vi "rsidr_core_global.vi"() -> ()   [LabVIEW 2015, in "Rohde&Schwarz CMXP GPRF.lvlib"] (continued)
ARB File All Names", "Data Type"=6, "Command"="SOUR:GPRF:GEN{instance}:SEQ:APO:WAV:ALL?", "Access"=0, "Range Table"="", "Read Callback"="", "Write Callback"="", "Supported Models"="", "Instrument Options"="", "Flags"=0, "Help"="Queries the names of the ARB files in the file pool.\n\nAvailable Repeated Capabilities:\ninstance: i0, i1, i2, i3, i4, i5, i6, i7, i8, i9, i10, i11, i12, i13, i14, i15, i16, i17, i18, i19, i20, i21, i22, i23, i24, i25, i26, i27, i28, i29, i30, i31, i32\r\n\nRemote-control command(s):\nSOURce:GPRF:GEN<i>:SEQuencer:APOol:WAVeform:ALL?"}, {"Level"=4, "Class Only"=FALSE, "Identifier"="RSCMXPGPRF_ATTR_HIDDEN_SEQUENCER_ARB_FILE_SAMPLE_RATE", "Descriptive Name"="Sequencer ARB File Sample Rate", "Data Type"=1, "Command"="SOUR:GPRF:GEN{instance}:SEQ:APO:SRAT?", "Access"=0, "Range Table"="", "Read Callback"="", "Write Callback"="", "Supported Models"="", "Instrument Options"="", "Flags"=8, "Help"="Queries the sample rate of the ARB file with the specified <Index>.\n\nAvailable Repeated Capabilities:\ninstance: i0, i1, i2, i3, i4, i5, i6, i7, i8, i9, i10, i11, i12, i13, i14, i15, i16, i17, i18, i19, i20, i21, i22, i23, i24, i25, i26, i27, i28, i29, i30, i31, i32\r\n\nRemote-control command(s):\nSOURce:GPRF:GEN<i>:SEQuencer:APOol:SRATe?"}, {"Level"=4, "Class Only"=FALSE, "Identifier"="RSCMXPGPRF_ATTR_SEQUENCER_ARB_FILE_ALL_SAMPLE_RATES", "Descriptive Name"="Sequencer ARB File All Sample Rates", "Data Type"=6, "Command"="SOUR:GPRF:GEN{instance}:SEQ:APO:SRAT:ALL?", "Access"=0, "Range Table"="", "Read Callback"="", "Write Callback"="", "Supported Models"="", "Instrument Options"="", "Flags"=0, "Help"="Queries the sample rates of the ARB files in the file pool.\n\nAvailable Repeated Capabilities:\ninstance: i0, i1, i2, i3, i4, i5, i6, i7, i8, i9, i10, i11, i12, i13, i14, i15, i16, i17, i18, i19, i20, i21, i22, i23, i24, i25, i26, i27, i28, i29, i30, i31, i32\r\n\nRemote-control command(s):\nSOURce:GPRF:GEN<i>:SEQuencer:APOol:SRATe:ALL?"}, {"Level"=4, "Class Only"=FALSE, "Identifier"="RSCMXPGPRF_ATTR_HIDDEN_SEQUENCER_ARB_FILE_NUMBER_OF_SAMPLES", "Descriptive Name"="Sequencer ARB File Number Of Samples", "Data Type"=0, "Command"="SOUR:GPRF:GEN{instance}:SEQ:APO:SAMP?", "Access"=0, "Range Table"="", "Read Callback"="", "Write Callback"="", "Supported Models"="", "Instrument Options"="", "Flags"=8, "Help"="Queries the number of samples in the ARB file with the specified <Index>.\n\nAvailable Repeated Capabilities:\ninstance: i0, i1, i2, i3, i4, i5, i6, i7, i8, i9, i10, i11, i12, i13, i14, i15, i16, i17, i18, i19, i20, i21, i22, i23, i24, i25, i26, i27, i28, i29, i30, i31, i32\r\n\nRemote-control command(s):\nSOURce:GPRF:GEN<i>:SEQuencer:APOol:SAMPles?"}, {"Level"=4, "Class Only"=FALSE, "Identifier"="RSCMXPGPRF_ATTR_SEQUENCER_ARB_FILE_ALL_NUMBERS_OF_SAMPLES", "Descriptive Name"="Sequencer ARB File All Numbers Of Samples", "Data Type"=6, "Command"="SOUR:GPRF:GEN{instance}:SEQ:APO:SAMP:ALL?", "Access"=0, "Range Table"="", "Read Callback"="", "Write Callback"="", "Supported Models"="", "Instrument Options"="", "Flags"=0, "Help"="Queries the numbers of samples in the ARB files of the file pool.\n\nAvailable Repeated Capabilities:\ninstance: i0, i1, i2, i3, i4, i5, i6, i7, i8, i9, i10, i11, i12, i13, i14, i15, i16, i17, i18, i19, i20, i21, i22, i23, i24, i25, i26, i27, i28, i29, i30, i31, i32\r\n\nRemote-control command(s):\nSOURce:GPRF:GEN<i>:SEQuencer:APOol:SAMPles:ALL?"}, {"Level"=4, "Class Only"=FALSE, "Identifier"="RSCMXPGPRF_ATTR_HIDDEN_SEQUENCER_ARB_FILE_DURATION", "Descriptive Name"="Sequencer ARB File Duration", "Data Type"=1, "Command"="SOUR:GPRF:GEN{instance}:SEQ:APO:DUR?", "Access"=0, "Range Table"="", "Read Callback"="", "Write Callback"="", "Supported Models"="", "Instrument Options"="", "Flags"=8, "Help"="Queries the duration of the ARB file with the specified <Index>.\n\nAvailable Repeated Capabilities:\ninstance: i0, i1, i2, i3, i4, i5, i6, i7, i8, i9, i10, i11, i12, i13, i14, i15, i16, i17, i18, i19, i20, i21, i22, i23, i24, i25, i26, i27, i28, i29, i30, i31, i32\r\n\nRemote-control command(s):\nSOURce:GPRF:GEN<i>:SEQuencer:APOol:DURation?"}, {"Level"=4, "Class Only"=FALSE, "Identifier"="RSCMXPGPRF_ATTR_SEQUENCER_ARB_FILE_ALL_DURATIONS", "Descriptive Name"="Sequencer ARB File All Durations", "Data Type"=6, "Command"="SOUR:GPRF:GEN{instance}:SEQ:APO:DUR:ALL?", "Access"=0, "Range Table"="", "Read Callback"="", "Write Callback"="", "Supported Models"="", "Instrument Options"="", "Flags"=0, "Help"="Queries the durations of the ARB files in the file pool.\n\nAvailable Repeated Capabilities:\ninstance: i0, i1, i2, i3, i4, i5, i6, i7, i8, i9, i10, i11, i12, i13, i14, i15, i16, i17, i18, i19, i20, i21, i22, i23, i24, i25, i26, i27, i28, i29, i30, i31, i32\r\n\nRemote-control command(s):\nSOURce:GPRF:GEN<i>:SEQuencer:APOol:DURation:ALL?"}, {"Level"=4, "Class Only"=FALSE, "Identifier"="RSCMXPGPRF_ATTR_HIDDEN_SEQUENCER_ARB_FILE_REQ_OPTIONS", "Descriptive Name"="Sequencer ARB File Req Options", "Data Type"=2, "Command"="SOUR:GPRF:GEN{instance}:SEQ:APO:ROPT?", "Access"=0, "Range Table"="", "Read Callback"="", "Write Callback"="", "Supported Models"="", "Instrument Options"="", "Flags"=8, "Help"="Queries the options required by the ARB file with the specified <Index>.\n\nAvailable Repeated Capabilities:\ninstance: i0, i1, i2, i3, i4, i5, i6, i7, i8, i9, i10, i11, i12, i13, i14, i15, i16, i17, i18, i19, i20, i21, i22, i23, i24, i25, i26, i27, i28, i29, i30, i31, i32\r\n\nRemote-control command(s):\nSOURce:GPRF:GEN<i>:SEQuencer:APOol:ROPTion?"}, {"Level"=4, "Class Only"=FALSE, "Identifier"="RSCMXPGPRF_ATTR_SEQUENCER_ARB_FILE_ALL_REQ_OPTIONS", "Descriptive Name"="Sequencer ARB File All Req Options", "Data Type"=6, "Command"="SOUR:GPRF:GEN{instance}:SEQ:APO:ROPT:ALL?", "Access"=0, "Range Table"="", "Read Callback"="", "Write Callback"="", "Supported Models"="", "Instrument Options"="", "Flags"=0, "Help"="Queries the options required by the ARB files in the file pool.\n\nAvailable Repeated Capabilities:\ninstance: i0, i1, i2, i3, i4, i5, i6, i7, i8, i9, i10, i11, i12, i13, i14, i15, i16, i17, i18, i19, i20, i21, i22, i23, i24, i25, i26, i27, i28, i29, i30, i31, i32\r\n\nRemote-control command(s):\nSOURce:GPRF:GEN<i>:SEQuencer:APOol:ROPTion:ALL?"}, {"Level"=4, "Class Only"=FALSE, "Identifier"="RSCMXPGPRF_ATTR_HIDDEN_SEQUENCER_ARB_FILE_PEAK_OFFSETS", "Descriptive Name"="Sequencer ARB File Peak Offsets", "Data Type"=1, "Command"="SOUR:GPRF:GEN{instance}:SEQ:APO:POFF?", "Access"=0, "Range Table"="", "Read Callback"="", "Write Callback"="", "Supported Models"="", "Instrument Options"="", "Flags"=8, "Help"="Queries the peak offset of the ARB file with the specified <Index>.\n\nAvailable Repeated Capabilities:\ninstance: i0, i1, i2, i3, i4, i5, i6, i7, i8, i9, i10, i11, i12, i13, i14, i15, i16, i17, i18, i19, i20, i21, i22, i23, i24, i25, i26, i27, i28, i29, i30, i31, i32\r\n\nRemote-control command(s):\nSOURce:GPRF:GEN<i>:SEQuencer:APOol:POFFset?"}, {"Level"=4, "Class Only"=FALSE, "Identifier"="RSCMXPGPRF_ATTR_SEQUENCER_ARB_FILE_ALL_PEAK_OFFSETS", "Descriptive Name"="Sequencer ARB File All Peak Offsets", "Data Type"=6, "Command"="SOUR:GPRF:GEN{instance}:SEQ:APO:POFF:ALL?", "Access"=0, "Range Table"="", "Read Callback"="", "Write Callback"="", "Supported Models"="", "Instrument Options"="", "Flags"=0, "Help"="Queries the peak offsets of the ARB files in the file pool.\n\nAvailable Repeated Capabilities:\ninstance: i0, i1, i2, i3, i4, i5, i6, i7, i8, i9, i10, i11, i12, i13, i14, i15, i16, i17, i18, i19, i20, i21, i22, i23, i24, i25, i26, i27, i28, i29, i30, i31, i32\r\n\nRemote-control command(s):\nSOURce:GPRF:GEN<i>:SEQuencer:APOol:POFFset:ALL?"}, {"Level"=4, "Class Only"=FALSE, "Identifier"="RSCMXPGPRF_ATTR_HIDDEN_SEQUENCER_ARB_FILE_PEAK_TO_AVG_RATIO", "Descriptive Name"="Sequencer ARB File Peak To Avg Ratio", "Data Type"=1, "Command"="SOUR:GPRF:GEN{instance}:SEQ:APO:PAR?", "Access"=0, "Range Table"="", "Read Callback"="", "Write Callback"="", "Supported Models"="", "Instrument Options"="", "Flags"=8, "Help"="Queries the peak to average ratio of the ARB file with the specified <Index>.\n\nAvailable Repeated Capabilities:\ninstance: i0, i1, i2, i3, i4, i5, i6, i7, i8, i9, i10, i11, i12, i13, i14, i15, i16, i17, i18, i19, i20, i21, i22, i23, i24, i25, i26, i27, i28, i29, i30, i31, i32\r\n\nRemote-control command(s):\nSOURce:GPRF:GEN<i>:SEQuencer:APOol:PARatio?"}, {"Level"=4, "Class Only"=FALSE, "Identifier"="RSCMXPGPRF_ATTR_SEQUENCER_ARB_FILE_ALL_PEAK_TO_AVG_RATIOS", "Descriptive Name"="Sequencer ARB File All Peak To Avg Ratios", "Data Type"=6, "Command"="SOUR:GPRF:GEN{instance}:SEQ:APO:PAR:ALL?", "Access"=0, "Range Table"="", "Read Callback"="", "Write Callback"="", "Supported Models"="", "Instrument Options"="", "Flags"=0, "Help"="Queries the peak to average ratios of the ARB files in the file pool.\n\nAvailable Repeated Capabilities:\ninstance: i0, i1, i2, i3, i4, i5, i6, i7, i8, i9, i10, i11, i12, i13, i14, i15, i16, i17, i18, i19, i20, i21, i22, i23, i24, i25, i26, i27, i28, i29, i30, i31, i32\r\n\nRemote-control command(s):\nSOURce:GPRF:GEN<i>:SEQuencer:APOol:PARatio:ALL?"}, {"Level"=4, "Class Only"=FALSE, "Identifier"="RSCMXPGPRF_ATTR_HIDDEN_SEQUENCER_ARB_FILE_CRC_PROTECTION", "Descriptive Name"="Sequencer ARB File CRC Protection", "Data Type"=0, "Command"="SOUR:GPRF:GEN{instance}:SEQ:APO:CRCP?", "Access"=0, "Range Table"="rsCmxpGprf_rngNoYesNav", "Read Callback"="", "Write Callback"="", "Supported Models"="", "Instrument Options"="", "Flags"=8, "Help"="Queries whether the ARB file with the specified <Index> contains a CRC checksum.\n\nAvailable Repeated Capabilities:\ninstance: i0, i1, i2, i3, i4, i5, i6, i7, i8, i9, i10, i11, i12, i13, i14, i15, i16, i17, i18, i19, i20, i21, i22, i23, i24, i25, i26, i27, i28, i29, i30, i31, i32\r\n\nRemote-control command(s):\nSOURce:GPRF:GEN<i>:SEQuencer:APOol:CRCProtect?"}, {"Level"=4, "Class Only"=FALSE, "Identifier"="RSCMXPGPRF_ATTR_SEQUENCER_ARB_FILE_ALL_CRC_PROTECTIONS", "Descriptive Name"="Sequencer ARB File All CRC Protections", "Data Type"=6, "Command"="SOUR:GPRF:GEN{instance}:SEQ:APO:CRCP:ALL?", "Access"=0, "Range Table"="", "Read Callback"="", "Write Callback"="", "Supported Models"="", "Instrument Options"="", "Flags"=0, "Help"="Queries whether the ARB files in the file pool contain CRC checksums.\n\nAvailable Repeated Capabilities:\ninstance: i0, i1, i2, i3, i4, i5, i6, i7, i8, i9, i10, i11, i12, i13, i14, i15, i16, i17, i18, i19, i20, i21, i22, i23, i24, i25, i26, i27, i28, i29, i30, i31, i32\r\n\nRemote-control command(s):\nSOURce:GPRF:GEN<i>:SEQuencer:APOol:CRCProtect:ALL?"}, {"Level"=4, "Class Only"=FALSE, "Identifier"="RSCMXPGPRF_ATTR_HIDDEN_SEQUENCER_ARB_FILE_RELIABILITY_INDICATOR", "Descriptive Name"="Sequencer ARB File Reliability Indicator", "Data Type"=0, "Command"="SOUR:GPRF:GEN{instance}:SEQ:APO:REL?", "Access"=0, "Range Table"="", "Read Callback"="", "Write Callback"="", "Supported Models"="", "Instrument Options"="", "Flags"=8, "Help"="Queries the reliability indicator for the ARB file with the specified <Index>.\n\nAvailable Repeated Capabilities:\ninstance: i0, i1, i2, i3, i4, i5, i6, i7, i8, i9, i10, i11, i12, i13, i14, i15, i16, i17, i18, i19, i20, i21, i22, i23, i24, i25, i26, i27, i28, i29, i30, i31, i32\r\n\nRemote-control command(s):\nSOURce:GPRF:GEN<i>:SEQuencer:APOol:RELiability?"}, {"Level"=4, "Class Only"=FALSE, "Identifier"="RSCMXPGPRF_ATTR_SEQUENCER_ARB_FILE_ALL_RELIABILITY_INDICATORS", "Descriptive Name"="Sequencer ARB File All Reliability Indicators", "Data Type"=6, "Command"="SOUR:GPRF:GEN{instance}:SEQ:APO:REL:ALL?", "Access"=0, "Range Table"="", "Read Callback"="", "Write Callback"="", "Supported Models"="", "Instrument Options"="", "Flags"=0, "Help"="Queries the reliability indicators for all ARB files in the file pool.\n\nAvailable Repeated Capabilities:\ninstance: i0, i1, i2, i3, i4, i5, i6, i7, i8, i9, i10, i11, i12, i13, i14, i15, i16, i17, i18, i19, i20, i21, i22, i23, i24, i25, i26, i27, i28, i29, i30, i31, i32\r\n\nRemote-control command(s):\nSOURce:GPRF:GEN<i>:SEQuencer:APOol:RELiability:ALL?"}, {"Level"=4, "Class Only"=FALSE, "Identifier"="RSCMXPGPRF_ATTR_HIDDEN_SEQUENCER_ARB_FILE_RELIABILITY_MESSAGE", "Descriptive Name"="Sequencer ARB File Reliability Message", "Data Type"=2, "Command"="SOUR:GPRF:GEN{instance}:SEQ:APO:RMES?", "Access"=0, "Range Table"="", "Read Callback"="", "Write Callback"="", "Supported Models"="", "Instrument Options"="", "Flags"=8, "Help"="Queries the reliability message for the ARB file with the specified <Index>.\n\nAvailable Repeated Capabilities:\ninstance: i0, i1, i2, i3, i4, i5, i6, i7, i8, i9, i10, i11, i12, i13, i14, i15, i16, i17, i18, i19, i20, i21, i22, i23, i24, i25, i26, i27, i28, i29, i30, i31, i32\r\n\nRemote-control command(s):\nSOURce:GPRF:GEN<i>:SEQuencer:APOol:RMESsage?"}, {"Level"=4, "Class Only"=FALSE, "Identifier"="RSCMXPGPRF_ATTR_SEQUENCER_ARB_FILE_ALL_RELIABILITY_MESSAGES", "Descriptive Name"="Sequencer ARB File All Reliability Messages", "Data Type"=6, "Command"="SOUR:GPRF:GEN{instance}:SEQ:APO:RMES:ALL?", "Access"=0, "Range Table"="", "Read Callback"="", "Write Callback"="", "Supported Models"="", "Instrument Options"="", "Flags"=0, "Help"="Queries the reliability messages for all ARB files in the file pool.\n\nAvailable Repeated Capabilities:\ninstance: i0, i1, i2, i3, i4, i5, i6, i7, i8, i9, i10, i11, i12, i13, i14, i15, i16, i17, i18, i19, i20, i21, i22, i23, i24, i25, i26, i27, i28, i29, i30, i31, i32\r\n\nRemote-control command(s):\nSOURce:GPRF:GEN<i>:SEQuencer:APOol:RMESsage:ALL?"}, {"Level"=4, "Class Only"=FALSE, "Identifier"="RSCMXPGPRF_ATTR_HIDDEN_SEQUENCER_ARB_FILE_PATH", "Descriptive Name"="Sequencer ARB File Path", "Data Type"=2, "Command"="SOUR:GPRF:GEN{instance}:SEQ:APO:PATH?", "Access"=0, "Range Table"="", "Read Callback"="", "Write Callback"="", "Supported Models"="", "Instrument Options"="", "Flags"=8, "Help"="Queries the path and file name of the ARB file with the specified <Index>.\n\nAvailable Repeated Capabilities:\ninstance: i0, i1, i2, i3, i4, i5, i6, i7, i8, i9, i10, i11, i12, i13, i14, i15, i16, i17, i18, i19, i20, i21, i22, i23, i24, i25, i26, i27, i28, i29, i30, i31, i32\r\n\nRemote-control command(s):\nSOURce:GPRF:GEN<i>:SEQuencer:APOol:PATH?"}, {"Level"=4, "Class Only"=FALSE, "Identifier"="RSCMXPGPRF_ATTR_SEQUENCER_ARB_FILE_ALL_PATHS", "Descriptive Name"="Sequencer ARB File All Paths", "Data Type"=6, "Command"="SOUR:GPRF:GEN{instance}:SEQ:APO:PATH:ALL?", "Access"=0, "Range Table"="", "Read Callback"="", "Write Callback"="", "Supported Models"="", "Instrument Options"="", "Flags"=0, "Help"="Queries the path and file name of the ARB files in the file pool.\n\nAvailable Repeated Capabilities:\ninstance: i0, i1, i2, i3, i4, i5, i6, i7, i8, i9, i10, i11, i12, i13, i14, i15, i16, i17, i18, i19, i20, i21, i22, i23, i24, i25, i26, i27, i28, i29, i30, i31, i32\r\n\nRemote-control command(s):\nSOURce:GPRF:GEN<i>:SEQuencer:APOol:PATH:ALL?"}, {"Level"=3, "Class Only"=TRUE, "Identifier"="", "Descriptive Name"="Dual Tone", "Data Type"=0, "Command"="", "Access"=0, "Range Table"="", "Read Callback"="", "Write Callback"="", "Supported Models"="", "Instrument Options"="", "Flags"=0, "Help"="Dual tone settings"}, {"Level"=4, "Class Only"=FALSE, "Identifier"="RSCMXPGPRF_ATTR_SEQUENCER_FREQUENCY_OFFSET", "Descriptive Name"="Sequencer Frequency Offset", "Data Type"=1, "Command"="SOUR:GPRF:GEN{instance}:SEQ:DTON:OFR{source}", "Access"=2, "Range Table"="rsCmxpGprf_rngSequencerFrequencyOffset", "Read Callback"="", "Write Callback"="", "Supported Models"="", "Instrument Options"="", "Flags"=0, "Help"="Selects a positive or negative offset frequency. The frequency of the modulated signal is equal to the generator frequency plus the offset.\n\nAvailable Repeated Capabilities:\ninstance: i0, i1, i2, i3, i4, i5, i6, i7, i8, i9, i10, i11, i12, i13, i14, i15, i16, i17, i18, i19, i20, i21, i22, i23, i24, i25, i26, i27, i28, i29, i30, i31, i32\r\nsource: s1, s2\r\n\nRemote-control command(s):\nSOURce:GPRF:GEN<i>:SEQuencer:DTONe:OFRequency<source>"}, {"Level"=4, "Class Only"=FALSE, "Identifier"="RSCMXPGPRF_ATTR_SEQUENCER_LEVEL_RATIO", "Descriptive Name"="Sequencer Level Ratio", "Data Type"=1, "Command"="SOUR:GPRF:GEN{instance}:SEQ:DTON:RAT", "Access"=2, "Range Table"="rsCmxpGprf_rngSequencerLevelRatio", "Read Callback"="", "Write Callback"="", "Supported Models"="", "Instrument Options"="", "Flags"=0, "Help"="Specifies the ratio in dB between the RMS levels of the two signals.\n\nAvailable Repeated Capabilities:\ninstance: i0, i1, i2, i3, i4, i5, i6, i7, i8, i9, i10, i11, i12, i13, i14, i15, i16, i17, i18, i19, i20, i21, i22, i23, i24, i25, i26, i27, i28, i29, i30, i31, i32\r\n\nRemote-control command(s):\nSOURce:GPRF:GEN<i>:SEQuencer:DTONe:RATio"}, {"Level"=3, "Class Only"=TRUE, "Identifier"="", "Descriptive Name"="List", "Data Type"=0, "Command"="", "Access"=0, "Range Table"="", "Read Callback"="", "Write Callback"="", "Supported Models"="", "Instrument Options"="", "Flags"=0, "Help"="Sequence list settings"}, {"Level"=4, "Class Only"=FALSE, "Identifier"="RSCMXPGPRF_ATTR_SEQUENCER_LIST_CREATE", "Descriptive Name"="Sequencer List Create", "Data Type"=0, "Command"="SOUR:GPRF:GEN{instance}:SEQ:LIST:CRE", "Access"=1, "Range Table"="", "Read Callback"="", "Write Callback"="", "Supported Models"="", "Instrument Options"="", "Flags"=0, "Help"="Deletes all entries of the sequencer list and creates the defined number of new entries with default settings.\n\nAvailable Repeated Capabilities:\ninstance: i0, i1, i2, i3, i4, i5, i6, i7, i8, i9, i10, i11, i12, i13, i14, i15, i16, i17, i18, i19, i20, i21, i22, i23, i24, i25, i26, i27, i28, i29, i30, i31, i32\r\n\nRemote-control command(s):\nSOURce:GPRF:GEN<i>:SEQuencer:LIST:CREate"}, {"Level"=4, "Class Only"=FALSE, "Identifier"="RSCMXPGPRF_ATTR_HIDDEN_QUERY_SEQUENCER_LIST_FREQUENCY", "Descriptive Name"="Query Sequencer List Frequency", "Data Type"=0, "Command"="SOUR:GPRF:GEN{instance}:SEQ:LIST:FREQ?", "Access"=0, "Range Table"="", "Read Callback"="", "Write Callback"="", "Supported Models"="", "Instrument Options"="", "Flags"=8, "Help"="Queries the RF generator frequency for the sequencer list entry with the selected <Index>.\n\nAvailable Repeated Capabilities:\ninstance: i0, i1, i2, i3, i4, i5, i6, i7, i8, i9, i10, i11, i12, i13, i14, i15, i16, i17, i18, i19, i20, i21, i22, i23, i24, i25, i26, i27, i28, i29, i30, i31, i32\r\n\nRemote-control command(s):\nSOURce:GPRF:GEN<i>:SEQuencer:LIST:FREQuency?"}, {"Level"=4, "Class Only"=FALSE, "Identifier"="RSCMXPGPRF_ATTR_SEQUENCER_LIST_FREQUENCY", "Descriptive Name"="Sequencer List Frequency", "Data Type"=6, "Command"="SOUR:GPRF:GEN{instance}:SEQ:LIST:FREQ", "Access"=1, "Range Table"="", "Read Callback"="", "Write Callback"="", "Supported Models"="", "Instrument Options"="", "Flags"=0, "Help"="Defines the RF generator frequency for the sequencer list entry with the selected <Index>.\n\nAvailable Repeated Capabilities:\ninstance: i0, i1, i2, i3, i4, i5, i6, i7, i8, i9, i10, i11, i12, i13, i14, i15, i16, i17, i18, i19, i20, i21, i22, i23, i24, i25, i26, i27, i28, i29, i30, i31, i32\r\n\nRemote-control command(s):\nSOURce:GPRF:GEN<i>:SEQuencer:LIST:FREQuency"}, {"Level"=4, "Class Only"=FALSE, "Identifier"="RSCMXPGPRF_ATTR_SEQUENCER_LIST_ALL_FREQUENCIES", "Descriptive Name"="Sequencer List All Frequencies", "Data Type"=6, "Command"="SOUR:GPRF:GEN{instance}:SEQ:LIST:FREQ:ALL", "Access"=2, "Range Table"="", "Read Callback"="", "Write Callback"="", "Supported Models"="", "Instrument Options"="", "Flags"=0, "Help"="Defines the RF generator frequencies for all sequencer list entries.\n\nAvailable Repeated Capabilities:\ninstance: i0, i1, i2, i3, i4, i5, i6, i7, i8, i9, i10, i11, i12, i13, i14, i15, i16, i17, i18, i19, i20, i21, i22, i23, i24, i25, i26, i27, i28, i29, i30, i31, i32\r\n\nRemote-control command(s):\nSOURce:GPRF:GEN<i>:SEQuencer:LIST:FREQuency:ALL"}, {"Level"=4, "Class Only"=FALSE, "Identifier"="RSCMXPGPRF_ATTR_HIDDEN_QUERY_SEQUENCER_LIST_LEVEL", "Descriptive Name"="Query Sequencer List Level", "Data Type"=0, "Command"="SOUR:GPRF:GEN{instance}:SEQ:LIST:LRMS?", "Access"=0, "Range Table"="", "Read Callback"="", "Write Callback"="", "Supported Models"="", "Instrument Options"="", "Flags"=8, "Help"="Queries the level for the sequencer list entry with the selected <Index>.\n\nAvailable Repeated Capabilities:\ninstance: i0, i1, i2, i3, i4, i5, i6, i7, i8, i9, i10, i11, i12, i13, i14, i15, i16, i17, i18, i19, i20, i21, i22, i23, i24, i25, i26, i27, i28, i29, i30, i31, i32\r\n\nRemote-control command(s):\nSOURce:GPRF:GEN<i>:SEQuencer:LIST:LRMS?"}, {"Level"=4, "Class Only"=FALSE, "Identifier"="RSCMXPGPRF_ATTR_SEQUENCER_LIST_LEVEL", "Descriptive Name"="Sequencer List Level", "Data Type"=6, "Command"="SOUR:GPRF:GEN{instance}:SEQ:LIST:LRMS", "Access"=1, "Range Table"="", "Read Callback"="", "Write Callback"="", "Supported Models"="", "Instrument Options"="", "Flags"=0, "Help"="Defines the level for the sequencer list entry with the selected <Index>.\n\nAvailable Repeated Capabilities:\ninstance: i0, i1, i2, i3, i4, i5, i6, i7, i8, i9, i10, i11, i12, i13, i14, i15, i16, i17, i18, i19, i20, i21, i22, i23, i24, i25, i26, i27, i28, i29, i30, i31, i32\r\n\nRemote-control command(s):\nSOURce:GPRF:GEN<i>:SEQuencer:LIST:LRMS"}, {"Level"=4, "Class Only"=FALSE, "Identifier"="RSCMXPGPRF_ATTR_SEQUENCER_LIST_ALL_LEVELS", "Descriptive Name"="Sequencer List All Levels", "Data Type"=6, "Command"="SOUR:GPRF:GEN{instance}:SEQ:LIST:LRMS:ALL", "Access"=2, "Range Table"="", "Read Callback"="", "Write Callback"="", "Supported Models"="", "Instrument Options"="", "Flags"=0, "Help"="Defines the level for all sequencer list entries.\n\nAvailable Repeated Capabilities:\ninstance: i0, i1, i2, i3, i4, i5, i6, i7, i8, i9, i10, i11, i12, i13, i14, i15, i16, i17, i18, i19, i20, i21, i22, i23, i24, i25, i26, i27, i28, i29, i30, i31, i32\r\n\nRemote-control command(s):\nSOURce:GPRF:GEN<i>:SEQuencer:LIST:LRMS:ALL"}, {"Level"=4, "Class Only"=FALSE, "Identifier"="RSCMXPGPRF_ATTR_HIDDEN_QUERY_SEQUENCER_LIST_DIGITAL_GAIN", "Descriptive Name"="Query Sequencer List Digital Gain", "Data Type"=1, "Command"="SOUR:GPRF:GEN{instance}:SEQ:LIST:DGA?", "Access"=0, "Range Table"="", "Read Callback"="", "Write Callback"="", "Supported Models"="", "Instrument Options"="", "Flags"=8, "Help"="Queries the digital gain for the sequencer list entry with the selected <Index>.\n\nAvailable Repeated Capabilities:\ninstance: i0, i1, i2, i3, i4, i5, i6, i7, i8, i9, i10, i11, i12, i13, i14, i15, i16, i17, i18, i19, i20, i21, i22, i23, i24, i25, i26, i27, i28, i29, i30, i31, i32\r\n\nRemote-control command(s):\nSOURce:GPRF:GEN<i>:SEQuencer:LIST:DGAin?"}, {"Level"=4, "Class Only"=FALSE, "Identifier"="RSCMXPGPRF_ATTR_SEQUENCER_LIST_DIGITAL_GAIN", "Descriptive Name"="Sequencer List Digital Gain", "Data Type"=6, "Command"="SOUR:GPRF:GEN{instance}:SEQ:LIST:DGA", "Access"=1, "Range Table"="", "Read Callback"="", "Write Callback"="", "Supported Models"="", "Instrument Options"="", "Flags"=0, "Help"="Defines the digital gain for the sequencer list entry with the selected <Index>.\n\nAvailable Repeated Capabilities:\ninstance: i0, i1, i2, i3, i4, i5, i6, i7, i8, i9, i10, i11, i12, i13, i14, i15, i16, i17, i18, i19, i20, i21, i22, i23, i24, i25, i26, i27, i28, i29, i30, i31, i32\r\n\nRemote-control command(s):\nSOURce:GPRF:GEN<i>:SEQuencer:LIST:DGAin"}, {"Level"=4, "Class Only"=FALSE, "Identifier"="RSCMXPGPRF_ATTR_SEQUENCER_LIST_ALL_DIGITAL_GAINS", "Descriptive Name"="Sequencer List All Digital Gains", "Data Type"=6, "Command"="SOUR:GPRF:GEN{instance}:SEQ:LIST:DGA:ALL", "Access"=2, "Range Table"="", "Read Callback"="", "Write Callback"="", "Supported Models"="", "Instrument Options"="", "Flags"=0, "Help"="Defines the digital gains for all sequencer list entries.\n\nAvailable Repeated Capabilities:\ninstance: i0, i1, i2, i3, i4, i5, i6, i7, i8, i9, i10, i11, i12, i13, i14, i15, i16, i17, i18, i19, i20, i21, i22, i23, i24, i25, i26, i27, i28, i29, i30, i31, i32\r\n\nRemote-control command(s):\nSOURce:GPRF:GEN<i>:SEQuencer:LIST:DGAin:ALL"}, {"Level"=4, "Class Only"=FALSE, "Identifier"="RSCMXPGPRF_ATTR_SEQUENCER_LIST_SIGNALS_CATALOG", "Descriptive Name"="Sequencer List Signals Catalog", "Data Type"=6, "Command"="SOUR:GPRF:GEN{instance}:SEQ:LIST:SIGN:CAT?", "Access"=0, "Range Table"="", "Read Callback"="", "Write Callback"="", "Supported Models"="", "Instrument Options"="", "Flags"=0, "Help"="Queries all available signal types. The available types depend on the ARB file pool.\n\nAvailable Repeated Capabilities:\ninstance: i0, i1, i2, i3, i4, i5, i6, i7, i8, i9, i10, i11, i12, i13, i14, i15, i16, i17, i18, i19, i20, i21, i22, i23, i24, i25, i26, i27, i28, i29, i30, i31, i32\r\n\nRemote-control command(s):\nSOURce:GPRF:GEN<i>:SEQuencer:LIST:SIGNal:CATalog?"}, {"Level"=4, "Class Only"=FALSE, "Identifier"="RSCMXPGPRF_ATTR_HIDDEN_QUERY_SEQUENCER_LIST_SIGNAL", "Descriptive Name"="Query Sequencer List Signal", "Data Type"=2, "Command"="SOUR:GPRF:GEN{instance}:SEQ:LIST:SIGN?", "Access"=0, "Range Table"="", "Read Callback"="", "Write Callback"="", "Supported Models"="", "Instrument Options"="", "Flags"=8, "Help"="Queries the signal type for the sequencer list entry with the selected <Index>.\n\nAvailable Repeated Capabilities:\ninstance: i0, i1, i2, i3, i4, i5, i6, i7, i8, i9, i10, i11, i12, i13, i14, i15, i16, i17, i18, i19, i20, i21, i22, i23, i24, i25, i26, i27, i28, i29, i30, i31, i32\r\n\nRemote-control command(s):\nSOURce:GPRF:GEN<i>:SEQuencer:LIST:SIGNal?"}, {"Level"=4, "Class Only"=FALSE, "Identifier"="RSCMXPGPRF_ATTR_SEQUENCER_LIST_SIGNAL", "Descriptive Name"="Sequencer List Signal", "Data Type"=6, "Command"="SOUR:GPRF:GEN{instance}:SEQ:LIST:SIGN", "Access"=1, "Range Table"="", "Read Callback"="", "Write Callback"="", "Supported Models"="", "Instrument Options"="", "Flags"=0, "Help"="Defines the signal type for the sequencer list entry with the selected <Index>.\n\nAvailable Repeated Capabilities:\ninstance: i0, i1, i2, i3, i4, i5, i6, i7, i8, i9, i10, i11, i12, i13, i14, i15, i16, i17, i18, i19, i20, i21, i22, i23, i24, i25, i26, i27, i28, i29, i30, i31, i32\r\n\nRemote-control command(s):\nSOURce:GPRF:GEN<i>:SEQuencer:LIST:SIGNal"}, {"Level"=4, "Class Only"=FALSE, "Identifier"="RSCMXPGPRF_ATTR_SEQUENCER_LIST_ALL_SIGNALS", "Descriptive Name"="Sequencer List All Signals", "Data Type"=6, "Command"="SOUR:GPRF:GEN{instance}:SEQ:LIST:SIGN:ALL", "Access"=2, "Range Table"="", "Read Callback"="", "Write Callback"="", "Supported Models"="", "Instrument Options"="", "Flags"=0, "Help"="Defines the signal types for all sequencer list entries.\n\nAvailable Repeated Capabilities:\ninstance: i0, i1, i2, i3, i4, i5, i6, i7, i8, i9, i10, i11, i12, i13, i14, i15, i16, i17, i18, i19, i20, i21, i22, i23, i24, i25, i26, i27, i28, i29, i30, i31, i32\r\n\nRemote-control command(s):\nSOURce:GPRF:GEN<i>:SEQuencer:LIST:SIGNal:ALL"}, {"Level"=4, "Class Only"=FALSE, "Identifier"="RSCMXPGPRF_ATTR_HIDDEN_SEQUENCER_LIST_SAMPLE_RATE", "Descriptive Name"="Sequencer List Sample Rate", "Data Type"=1, "Command"="SOUR:GPRF:GEN{instance}:SEQ:LIST:SRAT?", "Access"=0, "Range Table"="", "Read Callback"="", "Write Callback"="", "Supported Models"="", "Instrument Options"="", "Flags"=8, "Help"="Queries the sample rate for the sequencer list entry with the selected <Index>.\n\nAvailable Repeated Capabilities:\ninstance: i0, i1, i2, i3, i4, i5, i6, i7, i8, i9, i10, i11, i12, i13, i14, i15, i16, i17, i18, i19, i20, i21, i22, i23, i24, i25, i26, i27, i28, i29, i30, i31, i32\r\n\nRemote-control command(s):\nSOURce:GPRF:GEN<i>:SEQuencer:LIST:SRATe?"}, {"Level"=4, "Class Only"=FALSE, "Identifier"="RSCMXPGPRF_ATTR_SEQUENCER_LIST_ALL_SAMPLE_RATES", "Descriptive Name"="Sequencer List All Sample Rates", "Data Type"=6, "Command"="SOUR:GPRF:GEN{instance}:SEQ:LIST:SRAT:ALL?", "Access"=0, "Range Table"="", "Read Callback"="", "Write Callback"="", "Supported Models"="", "Instrument Options"="", "Flags"=0, "Help"="Queries the sample rates for all sequencer list entries.\n\nAvailable Repeated Capabilities:\ninstance: i0, i1, i2, i3, i4, i5, i6, i7, i8, i9, i10, i11, i12, i13, i14, i15, i16, i17, i18, i19, i20, i21, i22, i23, i24, i25, i26, i27, i28, i29, i30, i31, i32\r\n\nRemote-control command(s):\nSOURce:GPRF:GEN<i>:SEQuencer:LIST:SRATe:ALL?"}, {"Level"=4, "Class Only"=FALSE, "Identifier"="RSCMXPGPRF_ATTR_HIDDEN_QUERY_SEQUENCER_LIST_INCREMENT", "Descriptive Name"="Query Sequencer List Increment", "Data Type"=0, "Command"="SOUR:GPRF:GEN{instance}:SEQ:LIST:LINC?", "Access"=0, "Range Table"="rsCmxpGprf_rngListIncrement", "Read Callback"="", "Write Callback"="", "Supported Models"="", "Instrument Options"="", "Flags"=8, "Help"="Queries the list increment for the sequencer list entry with the selected <Index>.\n\nAvailable Repeated Capabilities:\ninstance: i0, i1, i2, i3, i4, i5, i6, i7, i8, i9, i10, i11, i12, i13, i14, i15, i16, i17, i18, i19, i20, i21, i22, i23, i24, i25, i26, i27, i28, i29, i30, i31, i32\r\n\nRemote-control command(s):\nSOURce:GPRF:GEN<i>:SEQuencer:LIST:LINCrement?"}, {"Level"=4, "Class Only"=FALSE, "Identifier"="RSCMXPGPRF_ATTR_SEQUENCER_LIST_INCREMENT", "Descriptive Name"="Sequencer List Increment", "Data Type"=6, "Command"="SOUR:GPRF:GEN{instance}:SEQ:LIST:LINC", "Access"=1, "Range Table"="", "Read Callback"="", "Write Callback"="", "Supported Models"="", "Instrument Options"="", "Flags"=0, "Help"="Defines the list increment for the sequencer list entry with the selected <Index>.\n\nAvailable Repeated Capabilities:\ninstance: i0, i1, i2, i3, i4, i5, i6, i7, i8, i9, i10, i11, i12, i13, i14, i15, i16, i17, i18, i19, i20, i21, i22, i23, i24, i25, i26, i27, i28, i29, i30, i31, i32\r\n\nRemote-control command(s):\nSOURce:GPRF:GEN<i>:SEQuencer:LIST:LINCrement"}, {"Level"=4, "Class Only"=FALSE, "Identifier"="RSCMXPGPRF_ATTR_SEQUENCER_LIST_ALL_INCREMENTS", "Descriptive Name"="Sequencer List All Increments", "Data Type"=6, "Command"="SOUR:GPRF:GEN{instance}:SEQ:LIST:LINC:ALL", "Access"=2, "Range Table"="", "Read Callback"="", "Write Callback"="", "Supported Models"="", "Instrument Options"="", "Flags"=0, "Help"="Defines the list increments for all sequencer list entries.\n\nAvailable Repeated Capabilities:\ninstance: i0, i1, i2, i3, i4, i5, i6, i7, i8, i9, i10, i11, i12, i13, i14, i15, i16, i17, i18, i19, i20, i21, i22, i23, i24, i25, i26, i27, i28, i29, i30, i31, i32\r\n\nRemote-control command(s):\nSOURce:GPRF:GEN<i>:SEQuencer:LIST:LINCrement:ALL"}, {"Level"=4, "Class Only"=FALSE, "Identifier"="RSCMXPGPRF_ATTR_HIDDEN_QUERY_SEQUENCER_LIST_INC_TRANSITION", "Descriptive Name"="Query Sequencer List Inc Transition", "Data Type"=0, "Command"="SOUR:GPRF:GEN{instance}:SEQ:LIST:ITR?", "Access"=0, "Range Table"="rsCmxpGprf_rngListIncTransition", "Read Callback"="", "Write Callback"="", "Supported Models"="", "Instrument Options"="", "Flags"=8, "Help"="Queries a condition for the transition to the next list entry, for the sequencer list entry with the selected <Index>.\n\nAvailable Repeated Capabilities:\ninstance: i0, i1, i2, i3, i4, i5, i6, i7, i8, i9, i10, i11, i12, i13, i14, i15, i16, i17, i18, i19, i20, i21, i22, i23, i24, i25, i26, i27, i28, i29, i30, i31, i32\r\n\nRemote-control command(s):\nSOURce:GPRF:GEN<i>:SEQuencer:LIST:ITRansition?"}, {"Level"=4, "Class Only"=FALSE, "Identifier"="RSCMXPGPRF_ATTR_SEQUENCER_LIST_INC_TRANSITION", "Descriptive Name"="Sequencer List Inc Transition", "Data Type"=6, "Command"="SOUR:GPRF:GEN{instance}:SEQ:LIST:ITR", "Access"=1, "Range Table"="", "Read Callback"="", "Write Callback"="", "Supported Models"="", "Instrument Options"="", "Flags"=0, "Help"="Defines a condition for the transition to the next list entry, for the sequencer list entry with the selected <Index>.\n\nAvailable Repeated Capabilities:\ninstance: i0, i1, i2, i3, i4, i5, i6, i7, i8, i9, i10, i11, i12, i13, i14, i15, i16, i17, i18, i19, i20, i21, i22, i23, i24, i25, i26, i27, i28, i29, i30, i31, i32\r\n\nRemote-control command(s):\nSOURce:GPRF:GEN<i>:SEQuencer:LIST:ITRansition"}, {"Level"=4, "Class Only"=FALSE, "Identifier"="RSCMXPGPRF_ATTR_SEQUENCER_LIST_ALL_INC_TRANSITIONS", "Descriptive Name"="Sequencer List All Inc Transitions", "Data Type"=6, "Command"="SOUR:GPRF:GEN{instance}:SEQ:LIST:ITR:ALL", "Access"=2, "Range Table"="", "Read Callback"="", "Write Callback"="", "Supported Models"="", "Instrument Options"="", "Flags"=0, "Help"="Defines or queries a condition for the transition to the next list entry, for all sequencer list entries.\n\nAvailable Repeated Capabilities:\ninstance: i0, i1, i2, i3, i4, i5, i6, i7, i8, i9, i10, i11, i12, i13, i14, i15, i16, i17, i18, i19, i20, i21, i22, i23, i24, i25, i26, i27, i28, i29, i30, i31, i32\r\n\nRemote-control command(s):\nSOURce:GPRF:GEN<i>:SEQuencer:LIST:ITRansition:ALL"}, {"Level"=4, "Class Only"=FALSE, "Identifier"="RSCMXPGPRF_ATTR_HIDDEN_QUERY_SEQUENCER_LIST_ARB_CYCLES", "Descriptive Name"="Query Sequencer List ARB Cycles", "Data Type"=0, "Command"="SOUR:GPRF:GEN{instance}:SEQ:LIST:ACYC?", "Access"=0, "Range Table"="rsCmxpGprf_rngARBCycles", "Read Callback"="", "Write Callback"="", "Supported Models"="", "Instrument Options"="", "Flags"=8, "Help"="Queries the number of ARB cycles for the sequencer list entry with the selected <Index>.\n\nAvailable Repeated Capabilities:\ninstance: i0, i1, i2, i3, i4, i5, i6, i7, i8, i9, i10, i11, i12, i13, i14, i15, i16, i17, i18, i19, i20, i21, i22, i23, i24, i25, i26, i27, i28, i29, i30, i31, i32\r\n\nRemote-control command(s):\nSOURce:GPRF:GEN<i>:SEQuencer:LIST:ACYCles?"}, {"Level"=4, "Class Only"=FALSE, "Identifier"="RSCMXPGPRF_ATTR_SEQUENCER_LIST_ARB_CYCLES", "Descriptive Name"="Sequencer List ARB Cycles", "Data Type"=6, "Command"="SOUR:GPRF:GEN{instance}:SEQ:LIST:ACYC", "Access"=1, "Range Table"="", "Read Callback"="", "Write Callback"="", "Supported Models"="", "Instrument Options"="", "Flags"=0, "Help"="Defines the number of ARB cycles for the sequencer list entry with the selected <Index>.\n\nAvailable Repeated Capabilities:\ninstance: i0, i1, i2, i3, i4, i5, i6, i7, i8, i9, i10, i11, i12, i13, i14, i15, i16, i17, i18, i19, i20, i21, i22, i23, i24, i25, i26, i27, i28, i29, i30, i31, i32\r\n\nRemote-control command(s):\nSOURce:GPRF:GEN<i>:SEQuencer:LIST:ACYCles"}, {"Level"=4, "Class Only"=FALSE, "Identifier"="RSCMXPGPRF_ATTR_SEQUENCER_LIST_ALL_ARB_CYCLES", "Descriptive Name"="Sequencer List All ARB Cycles", "Data Type"=6, "Command"="SOUR:GPRF:GEN{instance}:SEQ:LIST:ACYC:ALL", "Access"=2, "Range Table"="", "Read Callback"="", "Write Callback"="", "Supported Models"="", "Instrument Options"="", "Flags"=0, "Help"="Defines the ARB cycles for all sequencer list entries.\n\nAvailable Repeated Capabilities:\ninstance: i0, i1, i2, i3, i4, i5, i6, i7, i8, i9, i10, i11, i12, i13, i14, i15, i16, i17, i18, i19, i20, i21, i22, i23, i24, i25, i26, i27, i28, i29, i30, i31, i32\r\n\nRemote-control command(s):\nSOURce:GPRF:GEN<i>:SEQuencer:LIST:ACYCles:ALL"}, {"Level"=4, "Class Only"=FALSE, "Identifier"="RSCMXPGPRF_ATTR_HIDDEN_QUERY_SEQUENCER_LIST_DWELL_TIME", "Descriptive Name"="Query Sequencer List Dwell Time", "Data Type"=1, "Command"="SOUR:GPRF:GEN{instance}:SEQ:LIST:DTIM?", "Access"=0, "Range Table"="rsCmxpGprf_rngListModeDwellTime", "Read Callback"="", "Write Callback"="", "Supported Models"="", "Instrument Options"="", "Flags"=8, "Help"="Queries the dwell time for the sequencer list entry with the selected <Index>.\n\nAvailable Repeated Capabilities:\ninstance: i0, i1, i2, i3, i4, i5, i6, i7, i8, i9, i10, i11, i12, i13, i14, i15, i16, i17, i18, i19, i20, i21, i22, i23, i24, i25, i26, i27, i28, i29, i30, i31, i32\r\n\nRemote-control command(s):\nSOURce:GPRF:GEN<i>:SEQuencer:LIST:DTIMe?"}, {"Level"=4, "Class Only"=FALSE, "Identifier"="RSCMXPGPRF_ATTR_SEQUENCER_LIST_DWELL_TIME", "Descriptive Name"="Sequencer List Dwell Time", "Data Type"=6, "Command"="SOUR:GPRF:GEN{instance}:SEQ:LIST:DTIM", "Access"=1, "Range Table"="", "Read Callback"="", "Write Callback"="", "Supported Models"="", "Instrument Options"="", "Flags"=0, "Help"="Defines the dwell time for the sequencer list entry with the selected <Index>.\n\nAvailable Repeated Capabilities:\ninstance: i0, i1, i2, i3, i4, i5, i6, i7, i8, i9, i10, i11, i12, i13, i14, i15, i16, i17, i18, i19, i20, i21, i22, i23, i24, i25, i26, i27, i28, i29, i30, i31, i32\r\n\nRemote-control command(s):\nSOURce:GPRF:GEN<i>:SEQuencer:LIST:DTIMe"}, {"Level"=4, "Class Only"=FALSE, "Identifier"="RSCMXPGPRF_ATTR_SEQUENCER_LIST_ALL_DWELL_TIMES", "Descriptive Name"="Sequencer List All Dwell Times", "Data Type"=6, "Command"="SOUR:GPRF:GEN{instance}:SEQ:LIST:DTIM:ALL", "Access"=2, "Range Table"="", "Read Callback"="", "Write Callback"="", "Supported Models"="", "Instrument Options"="", "Flags"=0, "Help"="Defines the dwell times for all sequencer list entries.\n\nAvailable Repeated Capabilities:\ninstance: i0, i1, i2, i3, i4, i5, i6, i7, i8, i9, i10, i11, i12, i13, i14, i15, i16, i17, i18, i19, i20, i21, i22, i23, i24, i25, i26, i27, i28, i29, i30, i31, i32\r\n\nRemote-control command(s):\nSOURce:GPRF:GEN<i>:SEQuencer:LIST:DTIMe:ALL"}, {"Level"=4, "Class Only"=FALSE, "Identifier"="RSCMXPGPRF_ATTR_HIDDEN_SEQUENCER_LIST_TRANSITION_TIME", "Descriptive Name"="Sequencer List Transition Time", "Data Type"=1, "Command"="SOUR:GPRF:GEN{instance}:SEQ:LIST:TTIM?", "Access"=0, "Range Table"="rsCmxpGprf_rngSequencerListTransitionTime", "Read Callback"="", "Write Callback"="", "Supported Models"="", "Instrument Options"="", "Flags"=8, "Help"="Queries the transition time for the sequencer list entry with the selected <Index>.\n\nAvailable Repeated Capabilities:\ninstance: i0, i1, i2, i3, i4, i5, i6, i7, i8, i9, i10, i11, i12, i13, i14, i15, i16, i17, i18, i19, i20, i21, i22, i23, i24, i25, i26, i27, i28, i29, i30, i31, i32\r\n\nRemote-control command(s):\nSOURce:GPRF:GEN<i>:SEQuencer:LIST:TTIMe?"}, {"Level"=4, "Class Only"=FALSE, "Identifier"="RSCMXPGPRF_ATTR_SEQUENCER_LIST_ALL_TRANSITION_TIMES", "Descriptive Name"="Sequencer List All Transition Times", "Data Type"=6, "Command"="SOUR:GPRF:GEN{instance}:SEQ:LIST:TTIM:ALL?", "Access"=0, "Range Table"="", "Read Callback"="", "Write Callback"="", "Supported Models"="", "Instrument Options"="", "Flags"=0, "Help"="Queries the transition times for all sequencer list entries.\n\nAvailable Repeated Capabilities:\ninstance: i0, i1, i2, i3, i4, i5, i6, i7, i8, i9, i10, i11, i12, i13, i14, i15, i16, i17, i18, i19, i20, i21, i22, i23, i24, i25, i26, i27, i28, i29, i30, i31, i32\r\n\nRemote-control command(s):\nSOURce:GPRF:GEN<i>:SEQuencer:LIST:TTIMe:ALL?"}, {"Level"=4, "Class Only"=FALSE, "Identifier"="RSCMXPGPRF_ATTR_SEQUENCER_LIST_CURRENT_INDEX", "Descriptive Name"="Sequencer List Current Index", "Data Type"=0, "Command"="SOUR:GPRF:GEN{instance}:SEQ:LIST:IND", "Access"=2, "Range Table"="", "Read Callback"="", "Write Callback"="", "Supported Models"="", "Instrument Options"="", "Flags"=0, "Help"="Selects an entry of the sequencer list. Some other attributes use this setting.\n\nAvailable Repeated Capabilities:\ninstance: i0, i1, i2, i3, i4, i5, i6, i7, i8, i9, i10, i11, i12, i13, i14, i15, i16, i17, i18, i19, i20, i21, i22, i23, i24, i25, i26, i27, i28, i29, i30, i31, i32\r\n\nRemote-control command(s):\nSOURce:GPRF:GEN<i>:SEQuencer:LIST:INDex"}, {"Level"=4, "Class Only"=FALSE, "Identifier"="RSCMXPGPRF_ATTR_SEQUENCER_LIST_ENTRY_INSERT", "Descriptive Name"="Sequencer List Entry Insert", "Data Type"=0, "Command"="SOUR:GPRF:GEN{instance}:SEQ:LIST:ENTR:INS", "Access"=1, "Range Table"="", "Read Callback"="", "Write Callback"="", "Supported Models"="", "Instrument Options"="", "Flags"=0, "Help"="Inserts a new entry into the sequencer list, after the selected entry.\n\nAvailable Repeated Capabilities:\ninstance: i0, i1, i2, i3, i4, i5, i6, i7, i8, i9, i10, i11, i12, i13, i14, i15, i16, i17, i18, i19, i20, i21, i22, i23, i24, i25, i26, i27, i28, i29, i30, i31, i32\r\n\nRemote-control command(s):\nSOURce:GPRF:GEN<i>:SEQuencer:LIST:ENTRy:INSert"}, 
